vi "XML Format.vi"() -> ()   [LabVIEW 2020]
uses:
  <vilib>/Utility/xml.llb/Write to XML File(string).vi
panel:
  out "xml string":string
  in  "ID":cluster{"Nom":string, "Prénom":string, "Age":u8}
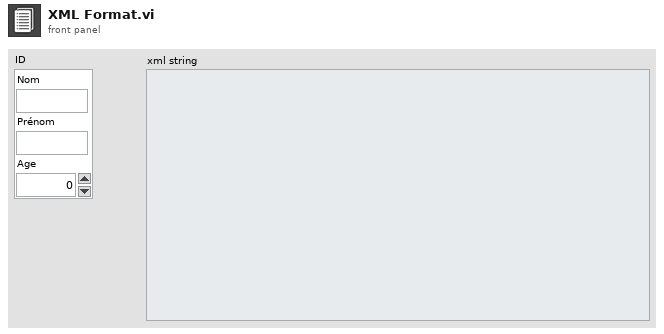
[diagram p1: front panel]
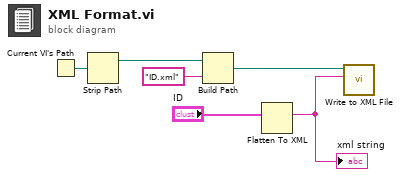
[diagram p0: block diagram]
diagram:
  n1 = Current VI's Path() -> (path=w5:path)
  n2 = Strip Path(path=w5) -> (stripped path=w4:path)  [unwired: 1 out]
  n3 = Build Path(base path=w4, name or relative path="ID.xml") -> (appended path=w2:path)
  n4 = Flatten To XML(6:"ID") -> (2:w1:string)
  "xml string" <- w1
  n5 = call-poly <vilib>:"Write to XML File.vi"("XML Input"=w1, "XML File Path"=w2) -> ()  [unwired: 7 in, 3 out]
